vi "Normalizer.vi"(8 "error in (no error)":errorcluster caption="entrée d'erreur (pas d'erreur)", 11 "Normalizer":cluster{"norm":string, "copy":bool}={"norm"="l2", "copy"=TRUE}) -> (0 "error out":errorcluster, 3 "Normalizer.lvclass":refnum<class "Normalizer.lvclass">)   [LabVIEW 2020]
doc: "Normalize samples individually to unit norm.\n\nEach sample (i.e. each row of the data matrix) with at least one non zero component is rescaled independently of other samples so that its norm (l1, l2 or inf) equals one.\n\nThis transformer is able to work both with dense numpy arrays and scipy.sparse matrix (use CSR format if you want to avoid the burden of a copy / conversion).\n\nScaling inputs to unit norms is a common operation for text classification or clustering for instance. For instance the dot product of two l2-normalized TF-IDF vectors is the cosine similarity of the vectors and is the base similarity metric for the Vector Space Model commonly used by the Information Retrieval community.\n\n\nParameters : \n\n- norm : ‘l1’, ‘l2’, or ‘max’, optional (‘l2’ by default)\nThe norm to use to normalize each non zero sample. If norm=’max’ is used, values will be rescaled by the maximum of the absolute values.\n\n- copy : boolean, optional, default True\nset to False to perform inplace row normalization and avoid a copy (if the input is already a numpy array or a scipy.sparse CSR matrix).\n\n\nMethods : \n\n- Fit : Do nothing and return the estimator unchanged. This method is just there to implement the usual API and hence work in pipelines.\n\nParameters : X : array-like\n\n\n- Fit Transform : Fit to data, then transform it. Fits transformer to X and y with optional parameters fit_params and returns a transformed version of X.\n\nParameters : X : {array-like, sparse matrix, dataframe} of shape (n_samples, n_features)\n y : ndarray of shape (n_samples,), default=None\n Target values.\n\nReturns : X_new : ndarray array of shape (n_samples, n_features_new)\n Transformed array.\n\n\n- Transform : Scale each non zero row of X to unit norm\n\nParameters : X : {array-like, sparse matrix}, shape [n_samples, n_features]\n The data to normalize, row by row. scipy.sparse matrices should be in CSR format to avoid an un-necessary copy."
uses:
  Normalizer.lvclass
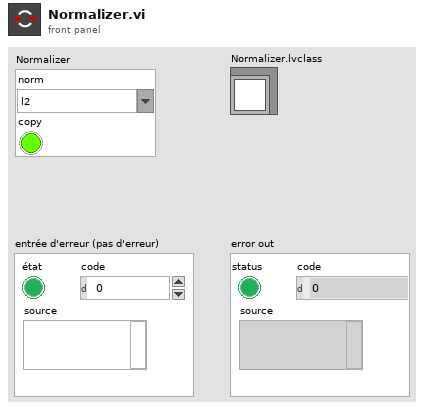
[diagram p1: front panel]
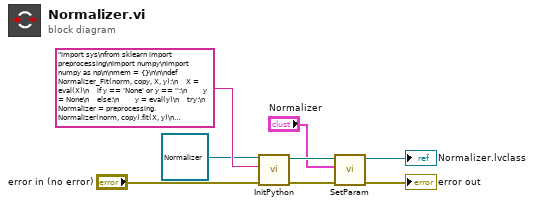
[diagram p0: block diagram]
diagram:
  n1 = call-dynamic "InitPython.vi"("error in (no error)"="error in (no error)", "Python Instruction"="import sys\nfrom sklearn import preprocessing\nimport numpy\nimport numpy as np\n\nmem = {}\n\n\ndef Normalizer_Fit(norm, copy, X, y):\n    X = eval(X)\n    if y == 'None' or y == '':\n        y = None\n    else:\n        y = eval(y)\n    try:\n        Normalizer = preprocessing.Normalizer(norm, copy).fit(X, y)\n        mem['FitNormalizer'] = Normalizer\n        return str('OK')\n    except:\n        erreur = sys.exc_info()\n        typerr = u\"%s\" % (erreur[0])\n        typerr = typerr[typerr.find(\"'\")+1:typerr.rfind(\"'\")]\n        msgerr = u\"%s\" % (erreur[1])\n        message = str('/!\\\\ {0} : {1}'. format(typerr,msgerr))\n        return message \n    \ndef Normalizer_FitTransform(norm, copy, X, y):\n    X = eval(X)\n    if y == 'None' or y == '':\n        y = None\n    else:\n        y = eval(y)\n    try:\n        Normalizer = preprocessing.Normalizer(norm, copy).fit_transform(X, y)\n        dtype = type(Normalizer)\n        if dtype == numpy.ndarray:\n            Normalizer = Normalizer.tolist()\n            return str(Normalizer) \n        else:\n            Mat = Normalizer.tocoo()\n            return str(list(zip(Mat.row, Mat.col, Mat.data)))\n    except:\n        erreur = sys.exc_info()\n        typerr = u\"%s\" % (erreur[0])\n        typerr = typerr[typerr.find(\"'\")+1:typerr.rfind(\"'\")]\n        msgerr = u\"%s\" % (erreur[1])\n        message = str('/!\\\\ {0} : {1}'. format(typerr,msgerr))\n        return message \n\ndef Normalizer_Transform(norm, copy, X, y):\n    X = eval(X)\n    if y == 'None' or y == '':\n        y = None\n    else:\n        y = eval(y)\n    try:\n        Normalizer = mem['FitNormalizer'].transform(X, y)\n        dtype = type(Normalizer)\n        if dtype == numpy.ndarray:\n            Normalizer = Normalizer.tolist()\n            return str(Normalizer) \n        else:\n            Mat = Normalizer.tocoo()\n            return str(list(zip(Mat.row, Mat.col, Mat.data)))\n    except:\n        erreur = sys.exc_info()\n        typerr = u\"%s\" % (erreur[0])\n        typerr = typerr[typerr.find(\"'\")+1:typerr.rfind(\"'\")]\n        msgerr = u\"%s\" % (erreur[1])\n        message = str('/!\\\\ {0} : {1}'. format(typerr,msgerr))\n        return message", "Scikit-learn en entrée"=refnum<class "Normalizer.lvclass"> refnum ("Normalizer.lvclass")) -> ("error out"=w4:errorcluster, "Scikit-learn en sortie"=w5:refnum<class "Normalizer.lvclass">)  [unwired: 7 in]
  n2 = call-dynamic "SetParam.vi"("error in (no error)"=w4, "Normalizer"="Normalizer", "Normalizer.lvclass"=w5) -> ("error out"=→"error out":errorcluster, "Normalizer.lvclass"=→"Normalizer.lvclass":refnum<class "Normalizer.lvclass">)  [unwired: 7 in]
